vi "Query and Display All FlexLogger Tags.vi"() -> ()   [LabVIEW 2020]
uses:
  <vilib>/Skyline/Tag/Wrapper/Wrapper AMQP_class/Query Tags AMQP.vi
  <vilib>/Skyline/Tag/Wrapper/Wrapper_class/Close Tag (Multiple).vi
  <vilib>/Skyline/Tag/Wrapper/Wrapper_class/NI Skyline Tag.lvclass
  <vilib>/Skyline/Tag/Wrapper/Wrapper AMQP_class/NI Skyline Tag AMQP.lvclass
  FlexLoggerTagHelpers.lvlib
panel:
  in  "Stop Button":bool
  in  "collect aggregates":bool
  out "Tags":i32[](listbox)
  # "Overview: This is example queries and displays all FlexLogger related tags\nRequirements: LabVIEW Full Development System, FlexLogger\nInstructions:\n1. Launch FlexLogger\n     a. Create a Project\n     b. Configure one or more channels in the Channel Specification\n     c. Using the Project >> Settings menu, enable Publish SystemLink Tags (Export) and Consume External SystemLink Tags (Import)\n     d. Restart the FlexLogger Project\n2. Run this VI\n3. Enable SystemLink metrics (max, min, mean) by clicking on collect aggregates.\n4. Note that tags exported by FlexLogger have Export in their path, and tags imported into FlexLogger have Import in their path."
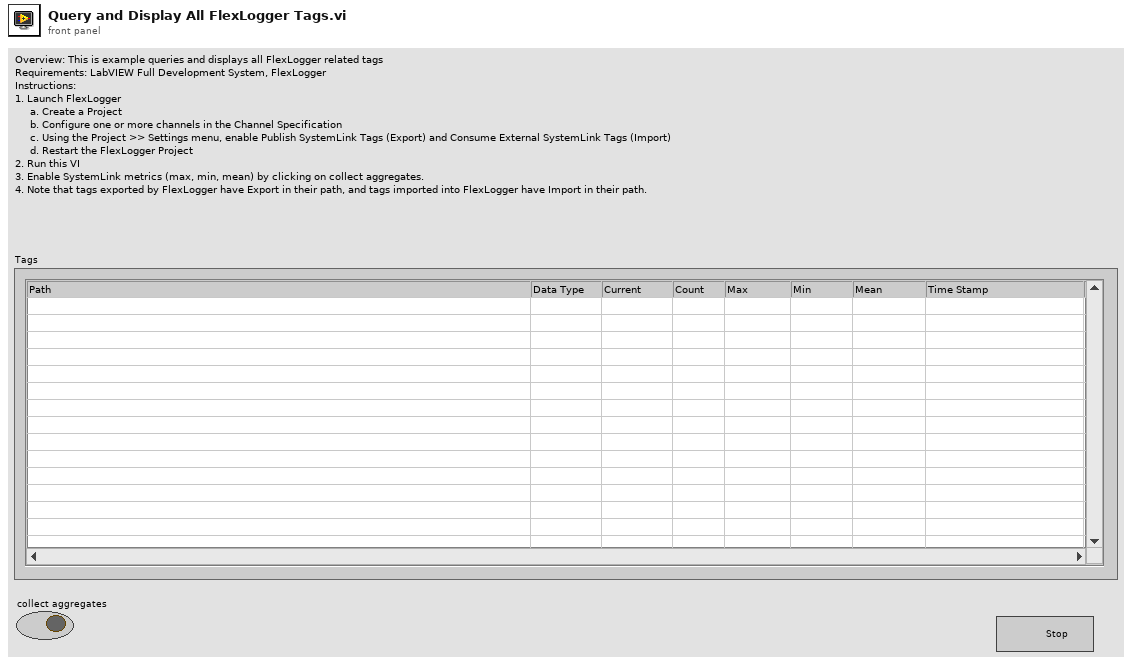
[diagram p1: front panel]
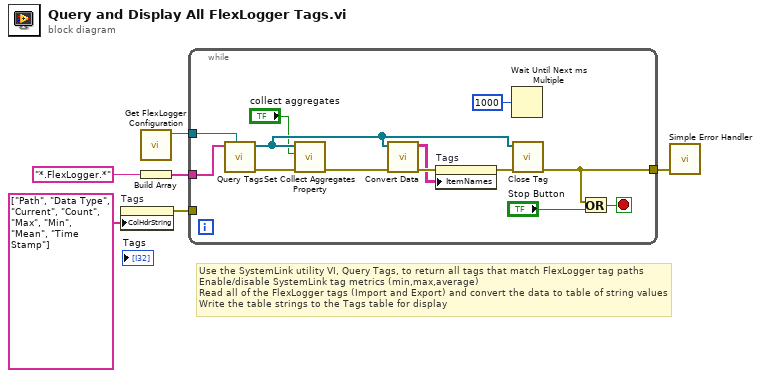
[diagram p0: block diagram]
diagram:
  # "Use the SystemLink utility VI, Query Tags, to return all tags that match FlexLogger tag paths\nEnable/disable SystemLink tag metrics (min,max,average)\nRead all of the FlexLogger tags (Import and Export) and convert the data to table of string values\nWrite the table strings to the Tags table for display"
  n1 = property on="Tags" class="MCListbox (strict)"("ColHdrString"=string[] ["Path", "Data Type", "Current", "Count", "Max", "Min", "Mean", "Time Stamp"] ("Row Header Strings[]")) -> (error out=w2:errorcluster)  [unwired: 2 in, 1 out]
  n2 = call "Get FlexLogger Configuration.vi"() -> ("Local FlexLogger Configuration"=w5:refnum<class "NI Skyline Configuration AMQP.lvclass">)  [unwired: 10 in, 1 out]
  n3 = Build Array("*.FlexLogger.*" ("namespace")) -> (w1:string[])
  n4 = while {
    tunnel: [w11] -> w6
    tunnel: w5 -> [w8]
    tunnel: w2 -> [_]
    tunnel: w1 -> [w7]
    stop <- w9 stop-if-true
    n5 = call-poly <vilib>:"Query Tags.vi"("configuration"=w8, "paths"=w7) -> ("error out"=w15:errorcluster, "tags"=w16:refnum<class "NI Skyline Tag.lvclass">[])  [unwired: 7 in, 1 out]
    n6 = call "Set Collect Aggregates Property.vi"("error in (no error)"=w15, "collect aggregates"="collect aggregates", "tags in"=w16) -> ("error out"=w14:errorcluster)  [unwired: 8 in]
    n7 = call "Convert Data.vi"("error in (no error)"=w14, "tags in"=w16) -> ("error out"=w18:errorcluster, "table of tag data"=w17:string[][])  [unwired: 8 in]
    n8 = property on="Tags" class="MCListbox (strict)"(error in=w18, "ItemNames"=w17) -> (error out=w19:errorcluster)  [unwired: 1 in, 1 out]
    n9 = Wait Until Next ms Multiple(millisecond multiple=u32 1000 ("milliseconds to wait")) -> ()  [unwired: 1 out]
    n10 = call-poly <vilib>:"Close Tag.vi"("error in (no error)"=w19, "tags"=w16) -> ("error out"=w11:errorcluster)  [unwired: 9 in]
    n11 = Or(x=w11, y="Stop Button") -> (x .or. y?=w9:bool)
  }
  n12 = call <vilib>:"Simple Error Handler.vi"("error in (no error)"=w6) -> ()  [unwired: 4 in, 5 out]
